vi "Generate Data.vi"(8 "Error In":errorcluster, 11 "Numeric Data In":refnum<class "Numeric Data.lvclass">) -> (0 "Error Out":errorcluster, 3 "Numeric Data Out":refnum<class "Numeric Data.lvclass">)   [LabVIEW 2022 SP3, in "Numeric Data.lvclass"]
doc: "This VI generates the numeric data."
uses:
  Numeric Data.lvclass
  <vilib>/numeric/Random Number (Range) DBL.vi
panel:
  out "Numeric Data":dbl
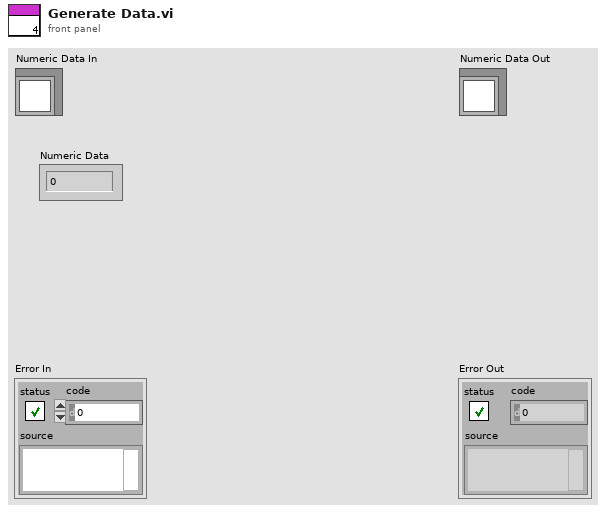
[diagram p1: front panel]
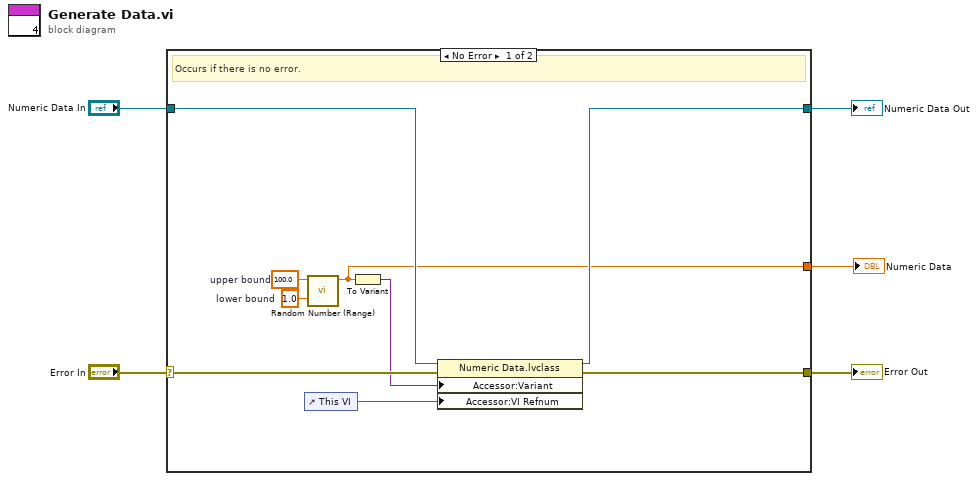
[diagram p0: block diagram]
diagram:
  n1 = case shown="No Error" "Error In" {
    selector: "Error In" -> [w14 w16]
    tunnel: [w9 w16] -> w4
    tunnel: [w8 w15] -> w2
    tunnel: "Numeric Data In" -> [w11 w15]
    tunnel: [w6 _] -> w1
    frame No Error {
      w12 = 1.0  # lower bound
      w13 = 100.0  # upper bound
      # "Occurs if there is no error."
      n2 = control-ref of="This VI"() -> (w7:refnum<vi>)
      n3 = call-poly <vilib>:"Random Number (Range).vi"("lower bound (0)"=w12, "upper bound (100)"=w13) -> ("number"=w6:dbl)  [unwired: 9 in]
      n4 = To Variant(anything=w6) -> (Variant=w10:variant)
      n5 = property class="Numeric Data.lvclass"(reference=w11, error in=w14, "Accessor:Variant"=w10, "Accessor:VI Refnum"=w7) -> (reference out=w8:refnum<class "Numeric Data.lvclass">, error out=w9:errorcluster)
    }
    frame Error {
      # "Occurs if there is any error."
    }
  }
  "Error Out" <- w4
  "Numeric Data Out" <- w2
  "Numeric Data" <- w1
